vi "Comparar precios.vi"(6 "Inventario":string, 8 "error in (no error)":errorcluster, 9 "Precio":string, 10 "Producto":string, 11 "UI Actor in":refnum<class "UI Actor.lvclass">) -> (0 "error out":errorcluster, 3 "UI Actor out":refnum<class "UI Actor.lvclass">)   [LabVIEW 2020, in "UI Actor.lvlib" / "UI Actor.lvclass"]
uses:
  UI Actor.lvclass
  UI Actor.lvclass/UI Actor.ctl
  Msg Messages/Update Msg Msg/Update Msg Msg.lvclass/Update Msg Msg.ctl
  <vilib>/ActorFramework/Message Enqueuer/Message Enqueuer.lvclass/Message Enqueuer.ctl
  Nestle  Actor Messages/Act Inventario Msg/Act Inventario Msg.lvclass/Act Inventario Msg.ctl
  <vilib>/ActorFramework/Message Enqueuer/Enqueue.vi
  Msg Messages/Update Msg Msg/Update Msg Msg.lvclass
  C:/Program Files (x86)/National Instruments/LabVIEW 2020/vi.lib/ActorFramework/Message/Message.lvclass
  Nestle  Actor Messages/Act Inventario Msg/Act Inventario Msg.lvclass
  Nestle  Actor Messages/Act Tabla Msg/Act Tabla Msg.lvclass
  <vilib>/ActorFramework/Message Priority Queue/Priority Enqueue.vi
  <vilib>/ActorFramework/Message Enqueuer/Message Enqueuer.lvclass
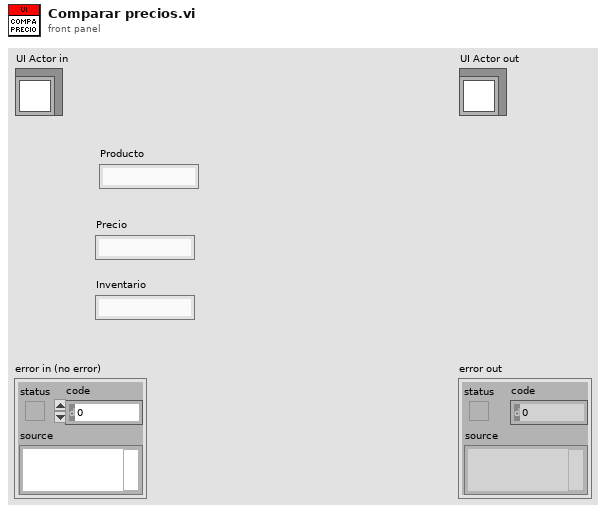
[diagram p1: front panel]
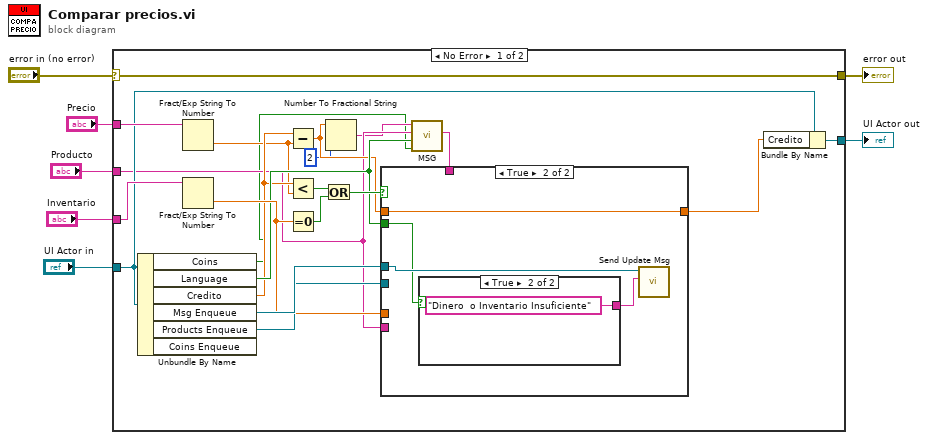
[diagram p0: block diagram]
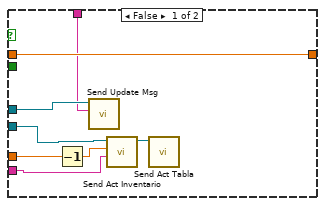
[diagram p2: hidden frame]
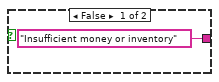
[diagram p3: hidden frame]
diagram:
  n1 = case shown="No Error" "error in (no error)" {
    selector: "error in (no error)" -> [w28 w44]
    tunnel: [w28 w44] -> w6
    tunnel: [w23 w43] -> w4
    tunnel: "UI Actor in" -> [w24 w43]
    tunnel: "Precio" -> [w26 _]
    tunnel: "Inventario" -> [w25 _]
    tunnel: "Producto" -> [w12 _]
    frame No Error {
      n2 = Unbundle By Name(w24) -> ("Coins"=w8:bool, "Language"=w17:bool, "Credito"=w15:dbl, "Msg Enqueue"=w27:refnum<class "Message Enqueuer.lvclass">, "Products Enqueue"=w22:refnum<class "Message Enqueuer.lvclass">)  [unwired: 1 out]
      n3 = Fract/Exp String To Number(string=w26) -> (number=w14:dbl)  [unwired: 3 in, 1 out]
      n4 = Fract/Exp String To Number(string=w25) -> (number=w18:dbl)  [unwired: 3 in, 1 out]
      n5 = Subtract(x=w15, y=w14) -> (x-y=w16:dbl)
      n6 = Less?(x=w15, y=w14) -> (x < y?=w20:bool)
      n7 = Equal To 0?(x=w18) -> (x = 0?=w19:bool)
      n8 = Or(x=w20, y=w19) -> (x .or. y?=w21:bool)
      n9 = Number To Fractional String(number=w16, precision (6)=i16 2) -> (F-format string=w11:string)  [unwired: 2 in]
      n10 = call "MSG.vi"("Coins"=w8, "Language"=w17, "Producto"=w12, "String"=w11) -> ("concatenated string"=w10:string)  [unwired: 7 in]
      n11 = case shown="True" w21 {
        tunnel: w18 -> [w36 _]
        tunnel: w27 -> [w35 w40]
        tunnel: w22 -> [w33 _]
        tunnel: w12 -> [w31 _]
        tunnel: w17 -> [_ w38]
        tunnel: w16 -> [w30 w37]
        tunnel: [w30 w37] -> w13
        tunnel: w10 -> [w29 _]
        frame False {
          n12 = Decrement(x=w36) -> (x-1=w34:dbl)
          n13 = call "Send Update Msg.vi"("Update Msg"=w29, "Message Enqueuer"=w35) -> ()  [unwired: 8 in, 2 out]
          n14 = call "Send Act Inventario.vi"("Producto"=w31, "Inventario"=w34, "Message Enqueuer"=w33) -> ("Message Enqueuer out"=w32:refnum<class "Message Enqueuer.lvclass">)  [unwired: 7 in, 1 out]
          n15 = call "Send Act Tabla.vi"("Message Enqueuer"=w32) -> ()  [unwired: 9 in, 2 out]
        }
        frame True {
          n16 = case shown="True" w38 {
            tunnel: ["Insufficient money or inventory" ("Update Msg") "Dinero  o Inventario Insuficiente" ("Update Msg")] -> w39
            frame False {
            }
            frame True {
            }
          }
          n17 = call "Send Update Msg.vi"("Update Msg"=w39, "Message Enqueuer"=w40) -> ()  [unwired: 8 in, 2 out]
        }
      }
      n18 = Bundle By Name(cluster=w24, "Credito"=w13) -> (w23:refnum<class "UI Actor.lvclass">)
    }
    frame Error {
    }
  }
  "error out" <- w6
  "UI Actor out" <- w4
